vi "CCDH_main.vi"() -> ()   [LabVIEW 2020]
panel:
  in  "L1":dbl
  out "T2":dbl
  out "T1":dbl
  out "L2":dbl
  out "L1":dbl
  out "LOAD_STATE":bool
  in  "stop":bool
  out "error out (no error)":errorcluster
  in  "error in (no error)":errorcluster
  in  "Chroma USB port":refnum<visa-resource-name>
  out "CURR":dbl
  out "VOLT":dbl
  out "error out (no error) 2":errorcluster
  in  "Path":path
  in  "Load":bool
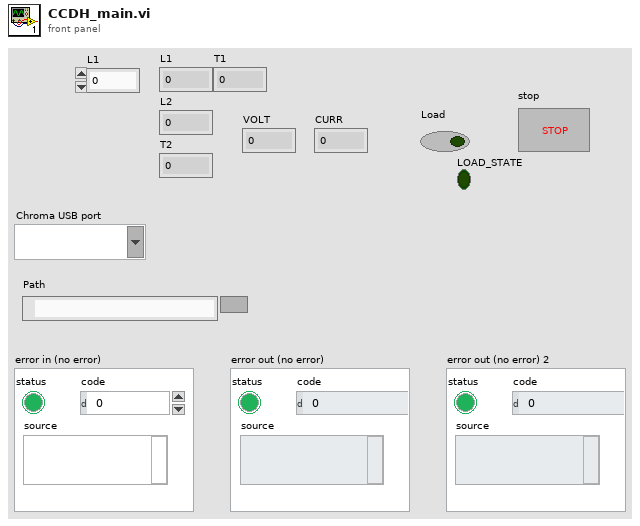
[diagram p1: front panel]
types:
  T1 = enum16{"open", "replace", "create", "open or create", "replace or create", "replace or create with confirmation"}
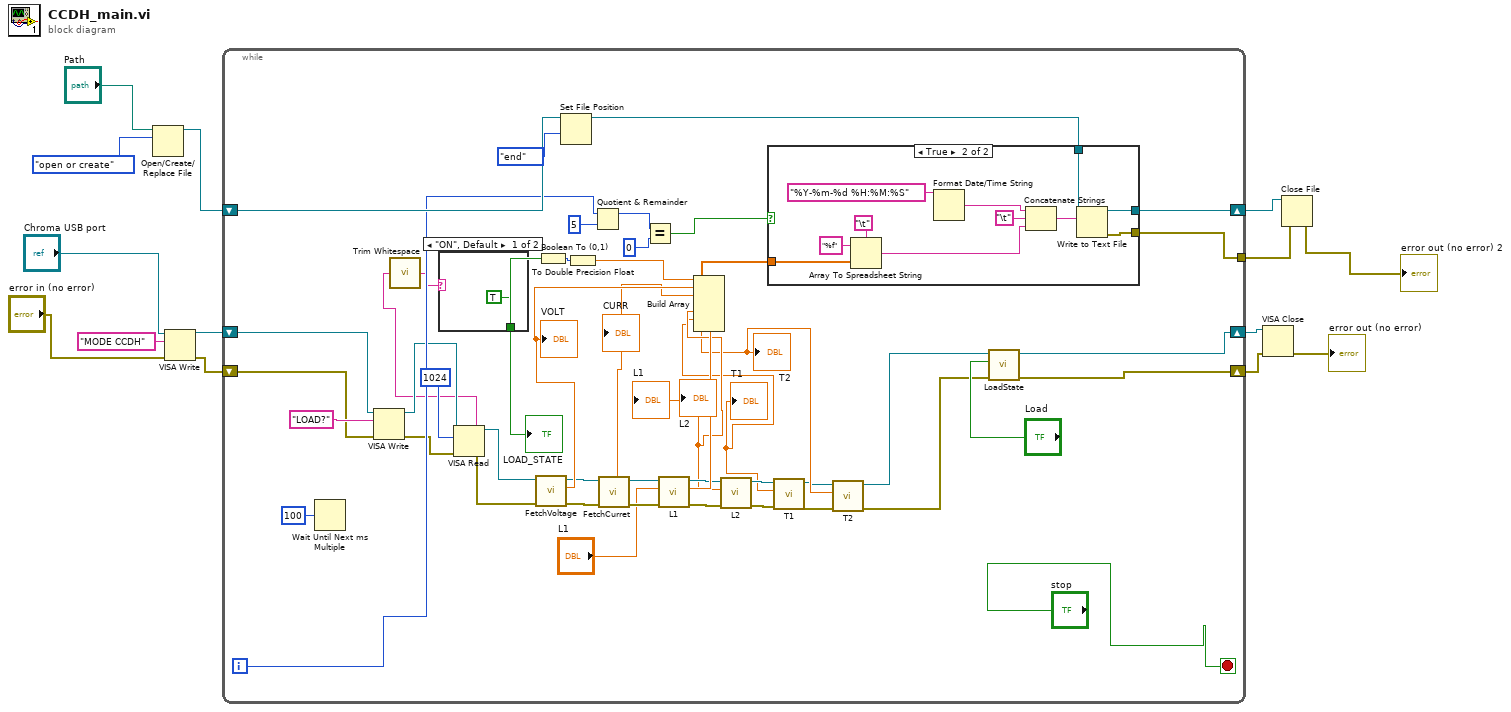
[diagram p0: block diagram]
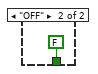
[diagram p2: hidden frame]
diagram:
  n1 = Open/Create/Replace File(file path (use dialog)="Path", operation (0:open)=T1."open or create") -> (refnum out=w9:refnum<file>)  [unwired: 4 in, 2 out]
  n2 = VISA Write(VISA resource name="Chroma USB port", write buffer="MODE CCDH", error in (no error)="error in (no error)") -> (VISA resource name out=w1:refnum<visa-resource-name>, error out=w3:errorcluster)  [unwired: 1 out]
  n3 = while {
    tunnel: [w61] -> w13
    shift-right: [w62] -> w14
    shift-left: w9 -> [w60]
    shift-right: [w35] -> w6
    shift-left: w1 -> [w42]
    shift-right: [w34] -> w7
    shift-left: w3 -> [w43]
    i -> [w45]
    stop <- "stop" stop-if-true
    n4 = Wait Until Next ms Multiple(millisecond multiple=u32 100) -> ()  [unwired: 1 out]
    n5 = VISA Write(VISA resource name=w42, write buffer="LOAD?", error in (no error)=w43) -> (VISA resource name out=w40:refnum<visa-resource-name>, error out=w38:errorcluster)  [unwired: 1 out]
    n6 = VISA Read(VISA resource name=w40, byte count=u32 1024, error in (no error)=w38) -> (VISA resource name out=w39:refnum<visa-resource-name>, read buffer=w32:string, error out=w37:errorcluster)  [unwired: 1 out]
    n7 = call <vilib>:"Trim Whitespace.vi"("string"=w32) -> ("trimmed string"=w31:string)  [unwired: 1 in]
    n8 = case shown="\"ON\", Default" w31 {
      tunnel: [TRUE FALSE] -> w33
      frame "ON", Default {
      }
      frame "OFF" {
      }
    }
    "LOAD_STATE" <- w33
    n9 = call "FetchVoltage.vi"("error in (no error)"=w37, "VISA Refnum in"=w39) -> ("error out"=w50:errorcluster, "Numeric"=w51:dbl, "VISA Refnum out"=w49:refnum<visa-resource-name>)  [unwired: 7 in]
    "VOLT" <- w51
    n10 = Boolean To (0,1)(Boolean=w33) -> (0, 1=w47:i16)
    n11 = Set File Position(refnum=w60, from (0:start)=enum16{"start", "end", "current"}."end") -> (refnum out=w55:refnum<file>)  [unwired: 2 in, 1 out]
    n12 = To Double Precision Float(number=w47) -> (double precision float=w46:dbl)
    n13 = Quotient & Remainder(x=w45, y=5) -> (x-y*floor(x/y)=w53:i32)  [unwired: 1 out]
    n14 = call "FetchCurret.vi"("error in (no error)"=w50, "VISA Refnum in"=w49) -> ("error out"=w29:errorcluster, "Numeric"=w48:dbl, "VISA Refnum out"=w30:refnum<visa-resource-name>)  [unwired: 7 in]
    "CURR" <- w48
    n15 = Equal?(x=w53, y=0) -> (x = y?=w58:bool)
    n16 = call "L1.vi"("error in (no error)"=w29, "Numeric"="L1", "VISA Refnum in"=w30) -> ("error out"=w26:errorcluster, "Numeric"=w28:dbl, "VISA Refnum out"=w27:refnum<visa-resource-name>)  [unwired: 6 in]
    "L1" <- w28
    n17 = call "L2.vi"("error in (no error)"=w26, "VISA Refnum in"=w27) -> ("error out"=w24:errorcluster, "Numeric"=w23:dbl, "VISA Refnum out"=w25:refnum<visa-resource-name>)  [unwired: 7 in]
    "L2" <- w23
    n18 = call "T1.vi"("error in (no error)"=w24, "VISA Refnum in"=w25) -> ("error out"=w17:errorcluster, "Numeric"=w22:dbl, "VISA Refnum out"=w18:refnum<visa-resource-name>)  [unwired: 7 in]
    "T1" <- w22
    n19 = call "T2.vi"("error in (no error)"=w17, "VISA Refnum in"=w18) -> ("error out"=w19:errorcluster, "Numeric"=w21:dbl, "VISA Refnum out"=w20:refnum<visa-resource-name>)  [unwired: 7 in]
    "T2" <- w21
    n20 = Build Array(w46, w51, w48, w28, w23, w22, w21) -> (w59:dbl[])
    n21 = case shown="True" w58 {
      tunnel: w59 -> [_ w74]
      tunnel: w55 -> [w65 w66]
      tunnel: [w65 w68] -> w62
      tunnel: [_ w67] -> w61
      frame False {
      }
      frame True {
        n22 = Array To Spreadsheet String(delimiter (Tab)="\t", array=w74, 3:"%f" ("format string")) -> (spreadsheet string=w71:string)
        n23 = Format Date/Time String(time format string (%c)="%Y-%m-%d %H:%M:%S") -> (date/time string=w72:string)  [unwired: 2 in]
        n24 = Concatenate Strings(w72, "\t", w71) -> (w69:string)
        n25 = Write to Text File(file (use dialog)=w66, text=w69) -> (refnum out=w68:refnum<file>, error out=w67:errorcluster)  [unwired: 2 in, 1 out]
      }
    }
    n26 = call "LoadState.vi"("error in (no error)"=w19, "Load"="Load", "VISA Refnum in"=w20) -> ("error out"=w34:errorcluster, "VISA Refnum out"=w35:refnum<visa-resource-name>)  [unwired: 7 in]
  }
  n27 = VISA Close(VISA resource name=w6, error in (no error)=w7) -> (error out=→"error out (no error)":errorcluster)
  n28 = Close File(refnum=w14, error in=w13) -> (error out=→"error out (no error) 2":errorcluster)  [unwired: 1 out]
